vi "Eulogy Date.vi"(8 "Error In":errorcluster, 10 "Tag Length":i32=5, 11 "Label Text":string) -> (0 "Error Out":errorcluster, 3 "Date":string)   [LabVIEW 2017, in "Bookmark Manager.lvlib"]
uses:
  Bookmark Manager.lvlib
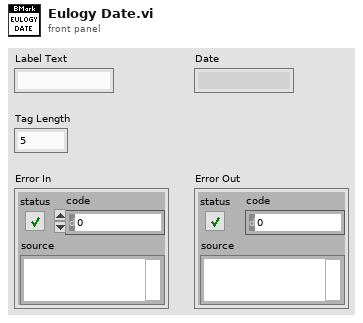
[diagram p1: front panel]
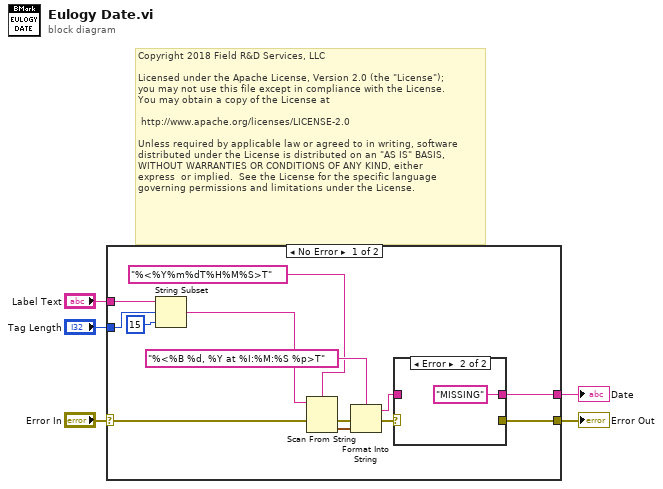
[diagram p0: block diagram]
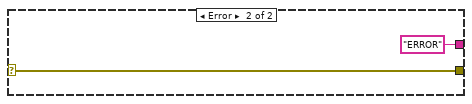
[diagram p3: hidden frame]
diagram:
  # "Copyright 2018 Field R&D Services, LLC\n\nLicensed under the Apache License, Version 2.0 (the \"License\");\nyou may not use this file except in compliance with the License.\nYou may obtain a copy of the License at\n\n\thttp://www.apache.org/licenses/LICENSE-2.0\n\nUnless required by applicable law or agreed to in writing, software\ndistributed under the License is distributed on an \"AS IS\" BASIS,\nWITHOUT WARRANTIES OR CONDITIONS OF ANY KIND, either \nexpress  or implied.  See the License for the specific language \ngoverning permissions and limitations under the License."
  n1 = case shown="No Error" "Error In" {
    selector: "Error In" -> [w10 w23]
    tunnel: [w6 "ERROR"] -> w5
    tunnel: [w8 w23] -> w4
    tunnel: "Label Text" -> [w13 _]
    tunnel: "Tag Length" -> [w11 _]
    frame No Error {
      n2 = String Subset(string=w13, offset (0)=w11, length (rest)=15 ("length (rest)")) -> (substring=w14:string)
      n3 = Scan From String(format string="%<%Y%m%dT%H%M%S>T", input string=w14, error in=w10) -> (error out=w16:errorcluster, output 1=w18:timestamp)  [unwired: 2 in, 2 out]
      n4 = Format Into String(format string="%<%B %d, %Y at %I:%M:%S %p>T", error in=w16, w18) -> (resulting string=w7:string, error out=w9:errorcluster)  [unwired: 1 in]
      n5 = case shown="Error" w9 {
        selector: w9 -> [w20 _]
        tunnel: [w20 _] -> w8
        tunnel: w7 -> [w19 _]
        tunnel: [w19 "MISSING"] -> w6
        frame No Error {
        }
        frame Error {
        }
      }
    }
    frame Error {
    }
  }
  "Date" <- w5
  "Error Out" <- w4
